vi "MDAQ_TargetSender.vi"(9 "Cluster IN":T1, 11 "Calibrated Graph":refnum<vi>) -> (1 "Cluster Out":T1)   [LabVIEW 2021]
uses:
  GUI_Def.ctl
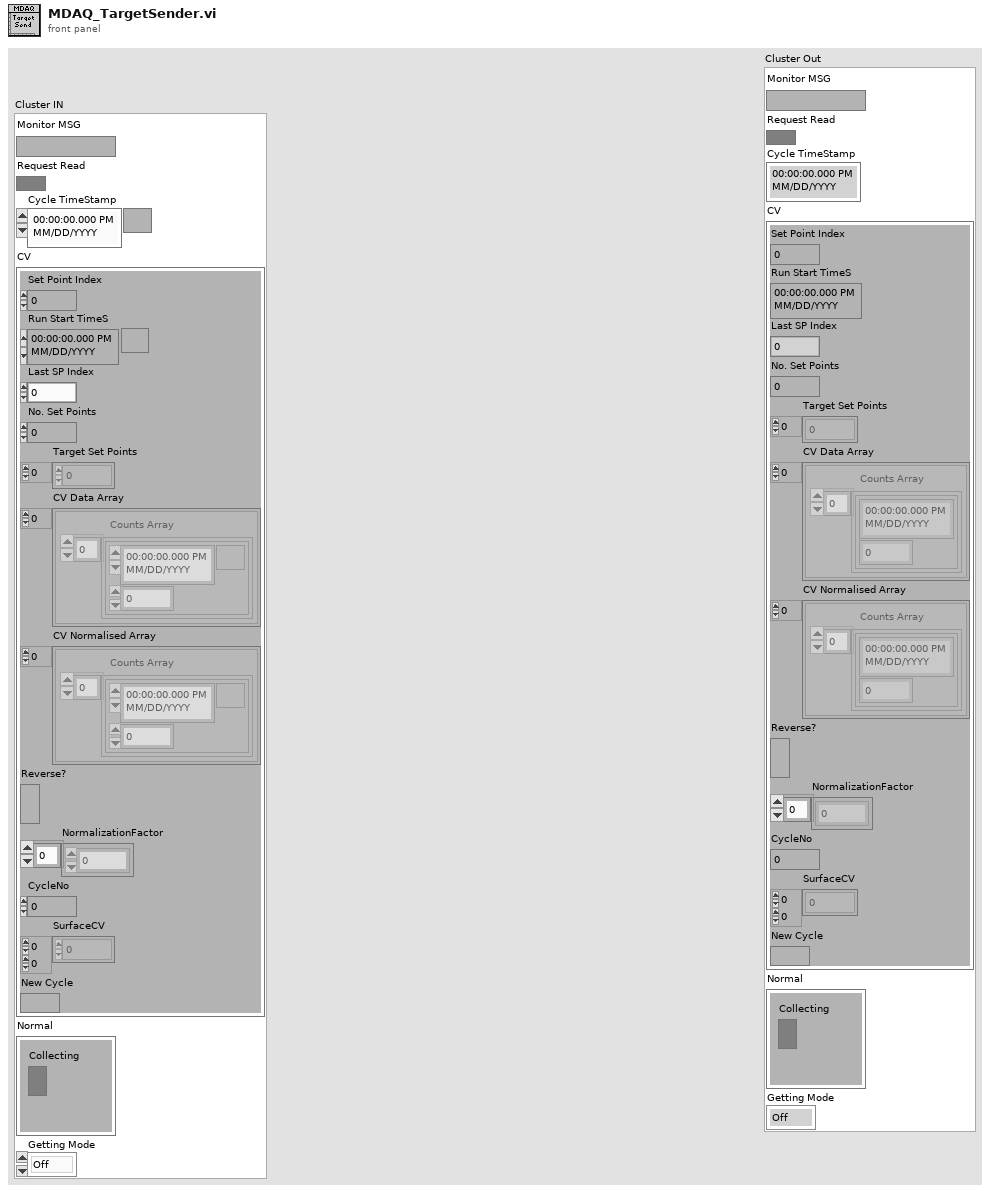
[diagram p1: front panel]
types:
  T1 = typedef "GUI_Def.ctl" = cluster{"Monitor MSG":string, "Request Read":bool, "Cycle TimeStamp":timestamp, "CV":cluster{"Set Point Index":u32, "Run Start TimeS":timestamp, "Last SP Index":u32, "No. Set Points":u32, "Target Set Points":dbl[], "CV Data Array":cluster{"Counts Array":cluster{timestamp, i32}[]}[], "CV Normalised Array":cluster{"Counts Array":cluster{timestamp, dbl}[]}[], "Reverse?":bool, "NormalizationFactor":i32[], "CycleNo":i32, "SurfaceCV":dbl[][], "New Cycle":bool}, "Normal":cluster{"Collecting":bool}, "Getting Mode":enum16{"Off", "Normal", "CV"}}
  T2 = typedef "LVCursorListTypeDef.ctl" = cluster{"Name":string, "Color":u32, "Style":u8, "Point Style":u8, "Name Visible":bool, "Allow Drag":bool, "Cursor Mode":u32, "Plot":i32, "Index":i32, "Position":cluster{"X":dbl, "Y":dbl}, "X Scale":u32, "Y Scale":u32, "Watch Plots":i32[], "Watch All Plots":bool, "Plot Area":i32, "Label Offset":cluster{"X":dbl, "Y":dbl}}[]
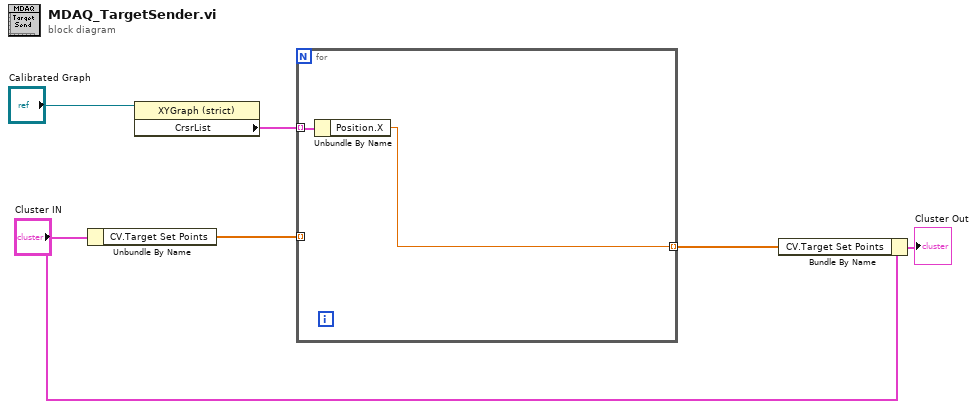
[diagram p0: block diagram]
diagram:
  n1 = Unbundle By Name("Cluster IN") -> ("CV.Target Set Points"=w6:dbl[])
  n2 = property class="XYGraph (strict)"(reference="Calibrated Graph") -> ("CrsrList"=w2:T2)  [unwired: 1 in, 2 out]
  n3 = for {
    tunnel: w6 -> [_] mode=indexing
    tunnel: w2 -> [w8] mode=indexing
    tunnel: [w7] -> w1 mode=indexing
    n4 = Unbundle By Name(w8) -> ("Position.X"=w7:dbl)
  }
  n5 = Bundle By Name(cluster="Cluster IN", "CV.Target Set Points"=w1) -> (→"Cluster Out":T1)
